vi "Write ERD Multiple Message Example.vi"(0 "GEA2 Reference In":refnum<k24>, 1 "Retry Count":i32=5, 2 "Read Timeout (ms)":u32=500, 5 "GEA Inputs":T2 {"Destination" format="%.0x"; "Source" format="%.0x"}, 7 "Write ERD List":T1[](array[typedef]) {"ERD Number" format="%.0x"}, 9 "Standalone?":bool=TRUE, 11 "Error In":errorcluster, 12 "#ERDs per message":i32=1 min=1 step=1, 13 "Verify ERD Response?":bool=TRUE) -> (4 "GEA2 Reference Out":refnum<k24>, 6 "Board ID":string, 8 "Raw Data Out":string[](array[string]), 15 "Error Out":errorcluster)   [LabVIEW 2014]
doc: "This is an example of how to use the GEA2 Write ERD multi-message VI. This VI splits up multiple ERD write requests into the number of messages you specify."
uses:
  C:/Automation/DLLs/PC Tools .NET/GeaCommunication.dll
  Automation/DLLs/PC Tools .NET/GeaCommunication.dll
  type defs/Source_Destination.ctl
  type defs/ERD Write Data In.ctl
  library/GEA2_Toolkit.lvlib
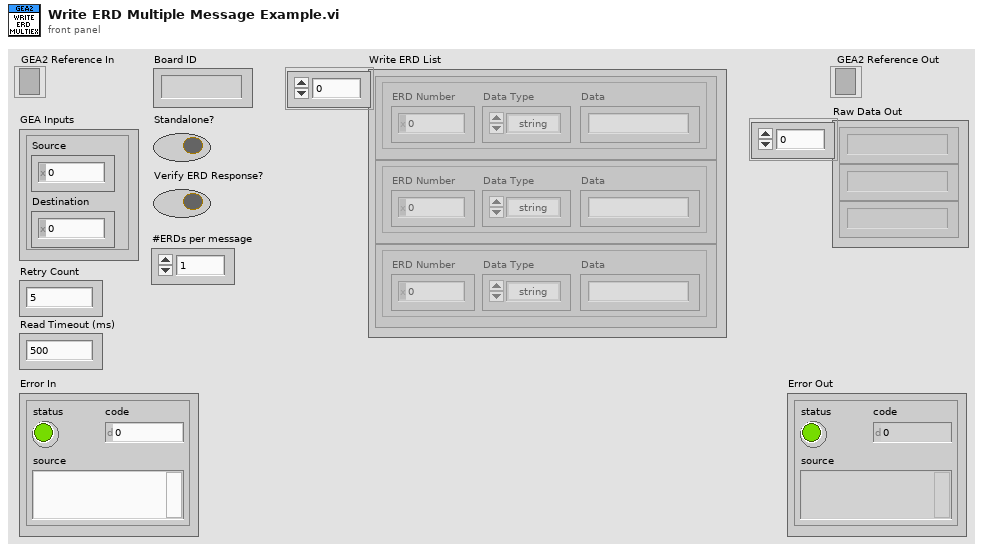
[diagram p1: front panel]
types:
  T1 = typedef "GEA2_Toolkit.lvlib/ERD Write Data In.ctl" = cluster{"ERD Number":u16, "Data Type":enum16{"string", "boolean", "uint8_t", "uint16_t", "uint32_t"}, "Data":string}
  T2 = typedef "GEA2_Toolkit.lvlib/Source_Destination.ctl" = cluster{"Source":u8, "Destination":u8}
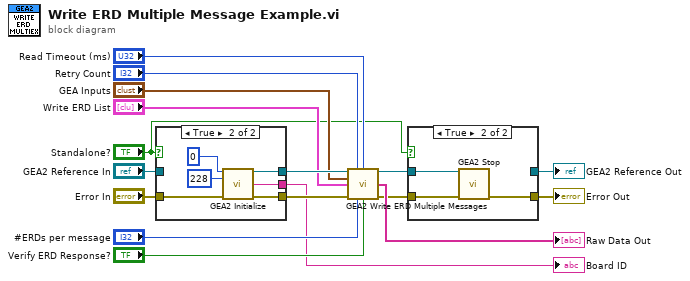
[diagram p0: block diagram]
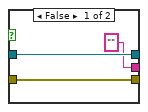
[diagram p3: hidden frame]
diagram:
  n1 = case shown="True" "Standalone?" {
    tunnel: [w19 w26] -> w14
    tunnel: "Error In" -> [w19 w25]
    tunnel: [w20 w22] -> w15
    tunnel: "GEA2 Reference In" -> [w20 _]
    tunnel: ["" ("Board ID") w21] -> w6
    frame False {
    }
    frame True {
      n2 = call "GEA2 Initialize.vi"("Board Index"=0, "Source Address"=u8 228, "error in"=w25) -> ("GEA2 Reference Out"=w22:refnum<k24>, "Board ID"=w21:string, "error out"=w26:errorcluster)  [unwired: 10 in]
    }
  }
  "Board ID" <- w6
  n3 = call "GEA2 Write ERD Multiple Messages.vi"("GEA2 Reference In"=w15, "Retry Count"="Retry Count", "Read Timeout (ms)"="Read Timeout (ms)", "GEA Inputs"="GEA Inputs", "Write ERD List"="Write ERD List", "Error In"=w14, "#ERDs per message"="#ERDs per message", "Verify ERD Response?"="Verify ERD Response?") -> ("GEA2 Reference Out"=w3:refnum<k24>, "Raw Data Out"=→"Raw Data Out":string[], "Error Out"=w4:errorcluster)  [unwired: 5 in]
  n4 = case shown="True" "Standalone?" {
    tunnel: [w28 w31] -> w5
    tunnel: w4 -> [w28 w30]
    tunnel: w3 -> [w27 w29]
    tunnel: [w27 _] -> w2
    frame False {
    }
    frame True {
      n5 = call "GEA2 Stop.vi"("GEA2 Reference In"=w29, "Error In"=w30) -> ("Error Out"=w31:errorcluster)  [unwired: 13 in]
    }
  }
  "Error Out" <- w5
  "GEA2 Reference Out" <- w2
